vi "波形发生器.vi"(2 "采样信息":cluster{"Fs":dbl, "#s":dbl}={"Fs"=1000.0, "#s"=1000.0} {"Fs" format="%.2p"}, 3 "formula":string="sin(w*t)*sin(2*pi(1)*t)" caption="公式", 4 "信噪比":dbl, 5 "square wave duty cycle (%)":dbl=50.0 caption="方波占空比(%)" format="%0.2f", 6 "相位":dbl format="%.2p", 7 "幅值":dbl=1.0 format="%0.2p", 8 "频率":dbl=10.0 format="%0.2p", 9 "停止":bool, 10 "噪声选择":enum16{"均匀白噪声", "高斯白噪声", "无"}(ring), 11 "波形选择":enum16{"公式波", "三角波", "方波", "正弦波"}(ring)) -> (1 "波形图":waveform(dbl)(graph))   [LabVIEW 2017]
uses:
  <vilib>/measure/NI_MABase.lvlib
  <vilib>/measure/NI_MAPro.lvlib
panel:
  # "波 形 发 生 器"
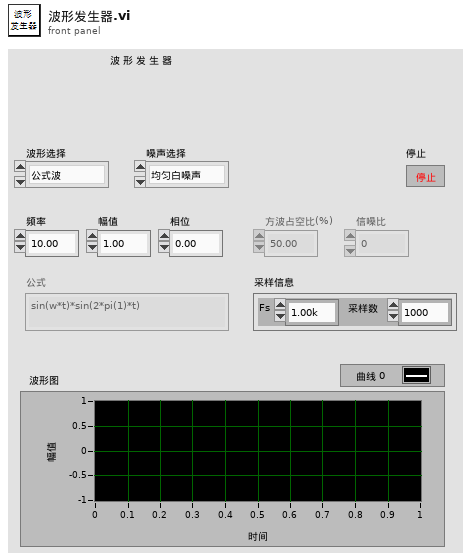
[diagram p1: front panel]
types:
  T1 = enum8{"Enabled", "Disabled", "Disabled and Grayed Out"}
  T2 = enum16{"Sine Wave", "Triangle Wave", "Square Wave", "Sawtooth Wave"}
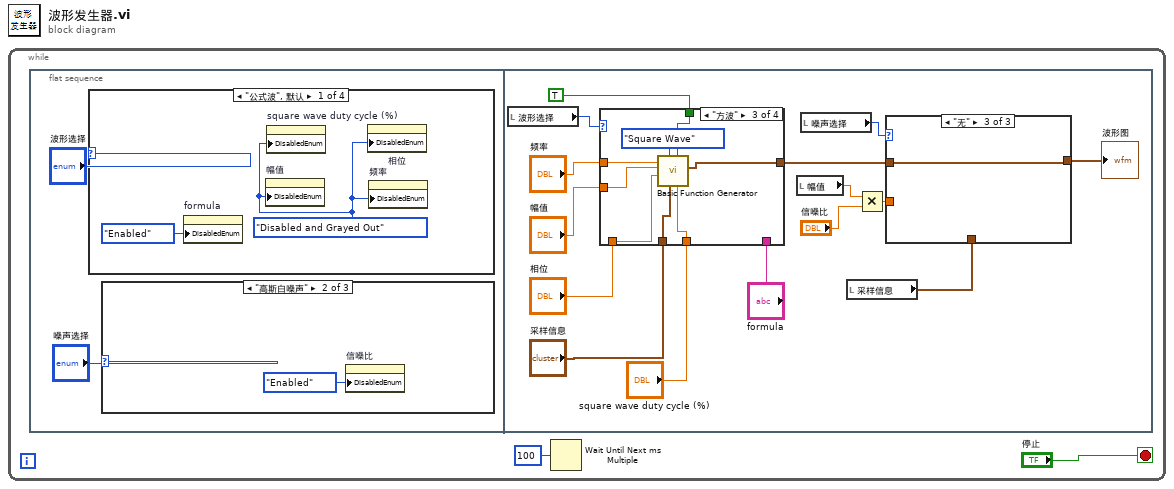
[diagram p0: block diagram]
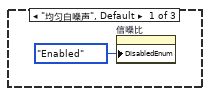
[diagram p2: hidden frame]
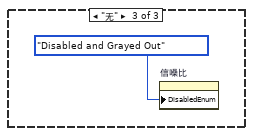
[diagram p3: hidden frame]
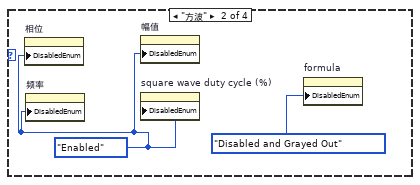
[diagram p4: hidden frame]
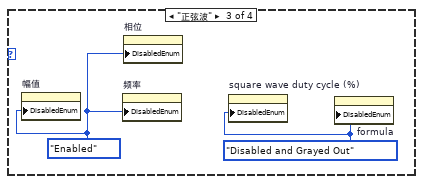
[diagram p5: hidden frame]
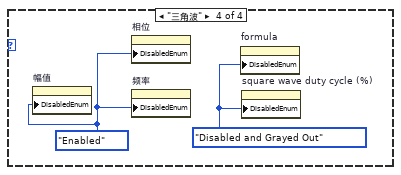
[diagram p6: hidden frame]
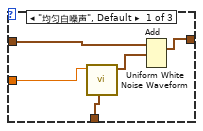
[diagram p7: hidden frame]
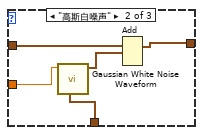
[diagram p8: hidden frame]
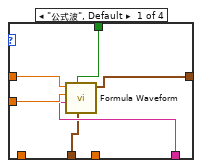
[diagram p9: hidden frame]
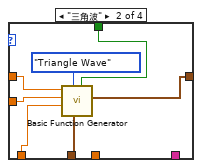
[diagram p10: hidden frame]
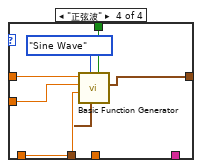
[diagram p11: hidden frame]
diagram:
  n1 = while {
    stop <- "停止" stop-if-true
    n2 = flat-sequence {
      frame #0 {
        n3 = case shown="\"公式波\", 默认" "波形选择" {
          frame "公式波", Default {
            w9 = T1."Disabled and Grayed Out" ("禁用")
            n4 = property on="formula" class="Str"("DisabledEnum"=T1."Enabled" ("禁用")) -> ()  [unwired: 2 in, 2 out]
            n5 = property on="幅值" class="DigNum (严格)"("DisabledEnum"=w9) -> ()  [unwired: 2 in, 2 out]
            n6 = property on="square wave duty cycle (%)" class="DigNum (严格)"("DisabledEnum"=w9) -> ()  [unwired: 2 in, 2 out]
            n7 = property on="相位" class="DigNum (严格)"("DisabledEnum"=w9) -> ()  [unwired: 2 in, 2 out]
            n8 = property on="频率" class="DigNum (严格)"("DisabledEnum"=w9) -> ()  [unwired: 2 in, 2 out]
          }
          frame "方波" {
            w10 = T1."Enabled" ("禁用")
            n9 = property on="相位" class="DigNum (严格)"("DisabledEnum"=w10) -> ()  [unwired: 2 in, 2 out]
            n10 = property on="频率" class="DigNum (严格)"("DisabledEnum"=w10) -> ()  [unwired: 2 in, 2 out]
            n11 = property on="幅值" class="DigNum (严格)"("DisabledEnum"=w10) -> ()  [unwired: 2 in, 2 out]
            n12 = property on="square wave duty cycle (%)" class="DigNum (严格)"("DisabledEnum"=w10) -> ()  [unwired: 2 in, 2 out]
            n13 = property on="formula" class="Str"("DisabledEnum"=T1."Disabled and Grayed Out" ("禁用")) -> ()  [unwired: 2 in, 2 out]
          }
          frame "正弦波" {
            w12 = T1."Enabled" ("禁用")
            w13 = T1."Disabled and Grayed Out" ("禁用")
            n14 = property on="幅值" class="DigNum (严格)"("DisabledEnum"=w12) -> ()  [unwired: 2 in, 2 out]
            n15 = property on="频率" class="DigNum (严格)"("DisabledEnum"=w12) -> ()  [unwired: 2 in, 2 out]
            n16 = property on="相位" class="DigNum (严格)"("DisabledEnum"=w12) -> ()  [unwired: 2 in, 2 out]
            n17 = property on="square wave duty cycle (%)" class="DigNum (严格)"("DisabledEnum"=w13) -> ()  [unwired: 2 in, 2 out]
            n18 = property on="formula" class="Str"("DisabledEnum"=w13) -> ()  [unwired: 2 in, 2 out]
          }
          frame "三角波" {
            w14 = T1."Enabled" ("禁用")
            w15 = T1."Disabled and Grayed Out" ("禁用")
            n19 = property on="幅值" class="DigNum (严格)"("DisabledEnum"=w14) -> ()  [unwired: 2 in, 2 out]
            n20 = property on="相位" class="DigNum (严格)"("DisabledEnum"=w14) -> ()  [unwired: 2 in, 2 out]
            n21 = property on="频率" class="DigNum (严格)"("DisabledEnum"=w14) -> ()  [unwired: 2 in, 2 out]
            n22 = property on="formula" class="Str"("DisabledEnum"=w15) -> ()  [unwired: 2 in, 2 out]
            n23 = property on="square wave duty cycle (%)" class="DigNum (严格)"("DisabledEnum"=w15) -> ()  [unwired: 2 in, 2 out]
          }
        }
        n24 = case shown="\"高斯白噪声\"" "噪声选择" {
          frame "均匀白噪声", Default {
            n25 = property on="信噪比" class="DigNum (严格)"("DisabledEnum"=T1."Enabled" ("禁用")) -> ()  [unwired: 2 in, 2 out]
          }
          frame "高斯白噪声" {
            n26 = property on="信噪比" class="DigNum (严格)"("DisabledEnum"=T1."Enabled" ("禁用")) -> ()  [unwired: 2 in, 2 out]
          }
          frame "无" {
            n27 = property on="信噪比" class="DigNum (严格)"("DisabledEnum"=T1."Disabled and Grayed Out" ("禁用")) -> ()  [unwired: 2 in, 2 out]
          }
        }
      }
      frame #1 {
        n28 = local read "波形选择"() -> (w30:enum16{"公式波", "三角波", "方波", "正弦波"})
        n29 = case shown="\"方波\"" w30 {
          tunnel: "频率" -> [w47 w52 w62 w69]
          tunnel: "幅值" -> [w46 w51 w61 w68]
          tunnel: "相位" -> [_ w50 w60 w67]
          tunnel: "采样信息" -> [w44 w54 w59 w66]
          tunnel: TRUE ("reset signal") -> [w43 w49 w57 w64]
          tunnel: "square wave duty cycle (%)" -> [_ _ w58 _]
          tunnel: "formula" -> [w45 _ _ _]
          tunnel: [w42 w48 w55 w63] -> w17
          frame "公式波", Default {
            n30 = call <vilib>:"Formula Waveform.vi"("sampling info"=w44, "reset signal"=w43, "formula"=w45, "amplitude"=w46, "frequency"=w47) -> ("signal out"=w42:waveform(dbl))  [unwired: 5 in, 1 out]
          }
          frame "三角波" {
            n31 = call <vilib>:"Basic Function Generator.vi"("reset signal"=w49, "sampling info"=w54, "signal type"=T2."Triangle Wave", "phase"=w50, "amplitude"=w51, "frequency"=w52) -> ("signal out"=w48:waveform(dbl))  [unwired: 3 in, 2 out]
          }
          frame "方波" {
            n32 = call <vilib>:"Basic Function Generator.vi"("square wave duty cycle (%)"=w58, "reset signal"=w57, "sampling info"=w59, "signal type"=T2."Square Wave", "phase"=w60, "amplitude"=w61, "frequency"=w62) -> ("signal out"=w55:waveform(dbl))  [unwired: 2 in, 2 out]
          }
          frame "正弦波" {
            n33 = call <vilib>:"Basic Function Generator.vi"("reset signal"=w64, "sampling info"=w66, "signal type"=T2."Sine Wave", "phase"=w67, "amplitude"=w68, "frequency"=w69) -> ("signal out"=w63:waveform(dbl))  [unwired: 3 in, 2 out]
          }
        }
        n34 = local read "幅值"() -> (w21:dbl)
        n35 = local read "噪声选择"() -> (w25:enum16{"均匀白噪声", "高斯白噪声", "无"})
        n36 = local read "采样信息"() -> (w18:cluster{"Fs":dbl, "#s":dbl})
        n37 = Multiply(x=w21, y="信噪比") -> (x*y=w19:dbl)
        n38 = case shown="\"无\"" w25 {
          tunnel: w19 -> [w35 w37 _]
          tunnel: w18 -> [w34 w36 _]
          tunnel: w17 -> [w33 w40 w41]
          tunnel: [w31 w38 w41] -> w16
          frame "均匀白噪声", Default {
            n39 = call <vilib>:"Uniform White Noise Waveform.vi"("sampling info"=w34, "amplitude"=w35) -> ("signal out"=w32:waveform(dbl))  [unwired: 8 in, 1 out]
            n40 = Add(1:w32, 2:w33) -> (0:w31:waveform(dbl))  [unwired: 1 in, 1 out]
          }
          frame "高斯白噪声" {
            n41 = call <vilib>:"Gaussian White Noise Waveform.vi"("sampling info"=w36, "standard deviation"=w37) -> ("signal out"=w39:waveform(dbl))  [unwired: 8 in, 1 out]
            n42 = Add(1:w39, 2:w40) -> (0:w38:waveform(dbl))  [unwired: 1 in, 1 out]
          }
          frame "无" {
          }
        }
        "波形图" <- w16
      }
    }
    n43 = Wait Until Next ms Multiple(millisecond multiple=u32 100 ("毫秒倍数")) -> ()  [unwired: 1 out]
  }
